vi "Thermistor (SubVI).vi"(11 "mean":dbl) -> (3 "T":dbl)   [LabVIEW 2023]
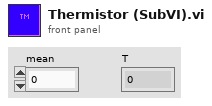
[diagram p1: front panel]
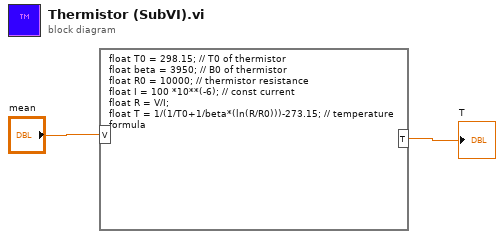
[diagram p0: block diagram]
diagram:
  n1 = formula code="float T0 = 298.15; // T0 of thermistor\nfloat beta = 3950; // B0 of thermistor\nfloat R0 = 10000; // thermistor resistance\nfloat I = 100 *10**(-6); // const current \nfloat R = V/I;\nfloat T = 1/(1/T0+1/beta*(ln(R/R0)))-273.15; // temperature formula"("V"="mean") -> ("T"=→"T":dbl)
